vi "Add CITI Package.vi"(8 "error in (no error)":errorcluster, 10 "CITI Package":T1, 11 "CITI reference in":refnum<k24>) -> (0 "error out":errorcluster, 3 "CITI reference out":refnum<k24>)   [LabVIEW 2023, in "NI_HFNetworkAnalysis.lvlib"]
doc: "Add a CITI package in memory for the specified CITI file.\n\n<b>Note</b>\nUse <b>Save CITI File.vi</b> to write all CITI packages in memory to the referenced CITI file."
uses:
  NI_HFNetworkAnalysis.lvlib
  C:/srd-semi-rfcal-software/AuxTools/STSRFFixtureCharactUtility/Source/Code Modules/Fixture/Dependencies/HFNetworkAnalysis/Support Files/NACE.Utils.Data.dll
  Support Files/NACE.Utils.Data.dll
  Controls/CITI Package.ctl
  <vilib>/Utility/VariantDataType/VariantType.lvlib
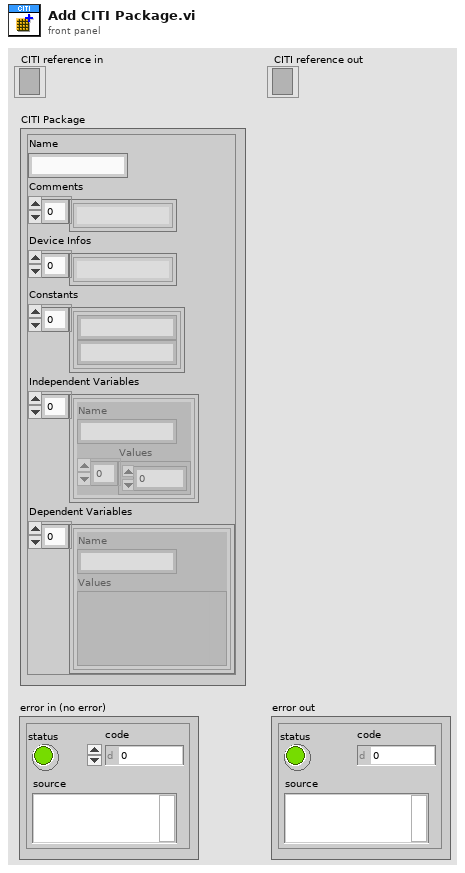
[diagram p1: front panel]
types:
  T1 = typedef "NI_HFNetworkAnalysis.lvlib/CITI Package.ctl" = cluster{"Name":string, "Comments":string[], "Device Infos":string[], "Constants":cluster{"Name":string, "Value":string}[], "Independent Variables":cluster{"Name":string, "Values":dbl[]}[], "Dependent Variables":cluster{"Name":string, "Values":variant}[]}
  T2 = typedef "VariantType.lvlib/Type.ctl" = enum8{"Invalid Type", "Void", "I8", "I16", "I32", "I64", "U8", "U16", "U32", "U64", "Single Float", "Double Float", "Extended Float", "Single Complex", "Double Complex", "Extended Complex", "Enum U8", "Enum U16", "Enum U32", "Enum U64", "Single Float With Unit", "Double Float With Unit", "Extended Float With Unit", "Single Complex with Unit", "Double Complex with Unit", "Extended Complex with Unit", "Boolean", "String", "Path", "Picture", "Tag", "Array", "Cluster", "Variant", "LV Variant", "Waveform", "Timestamp", "Digital Waveform", "Digital Data", "ExpressData", "Refnum", "External Data", "VI", "Poly VI", "LabVIEW Class Instance", "Fixed Point"}
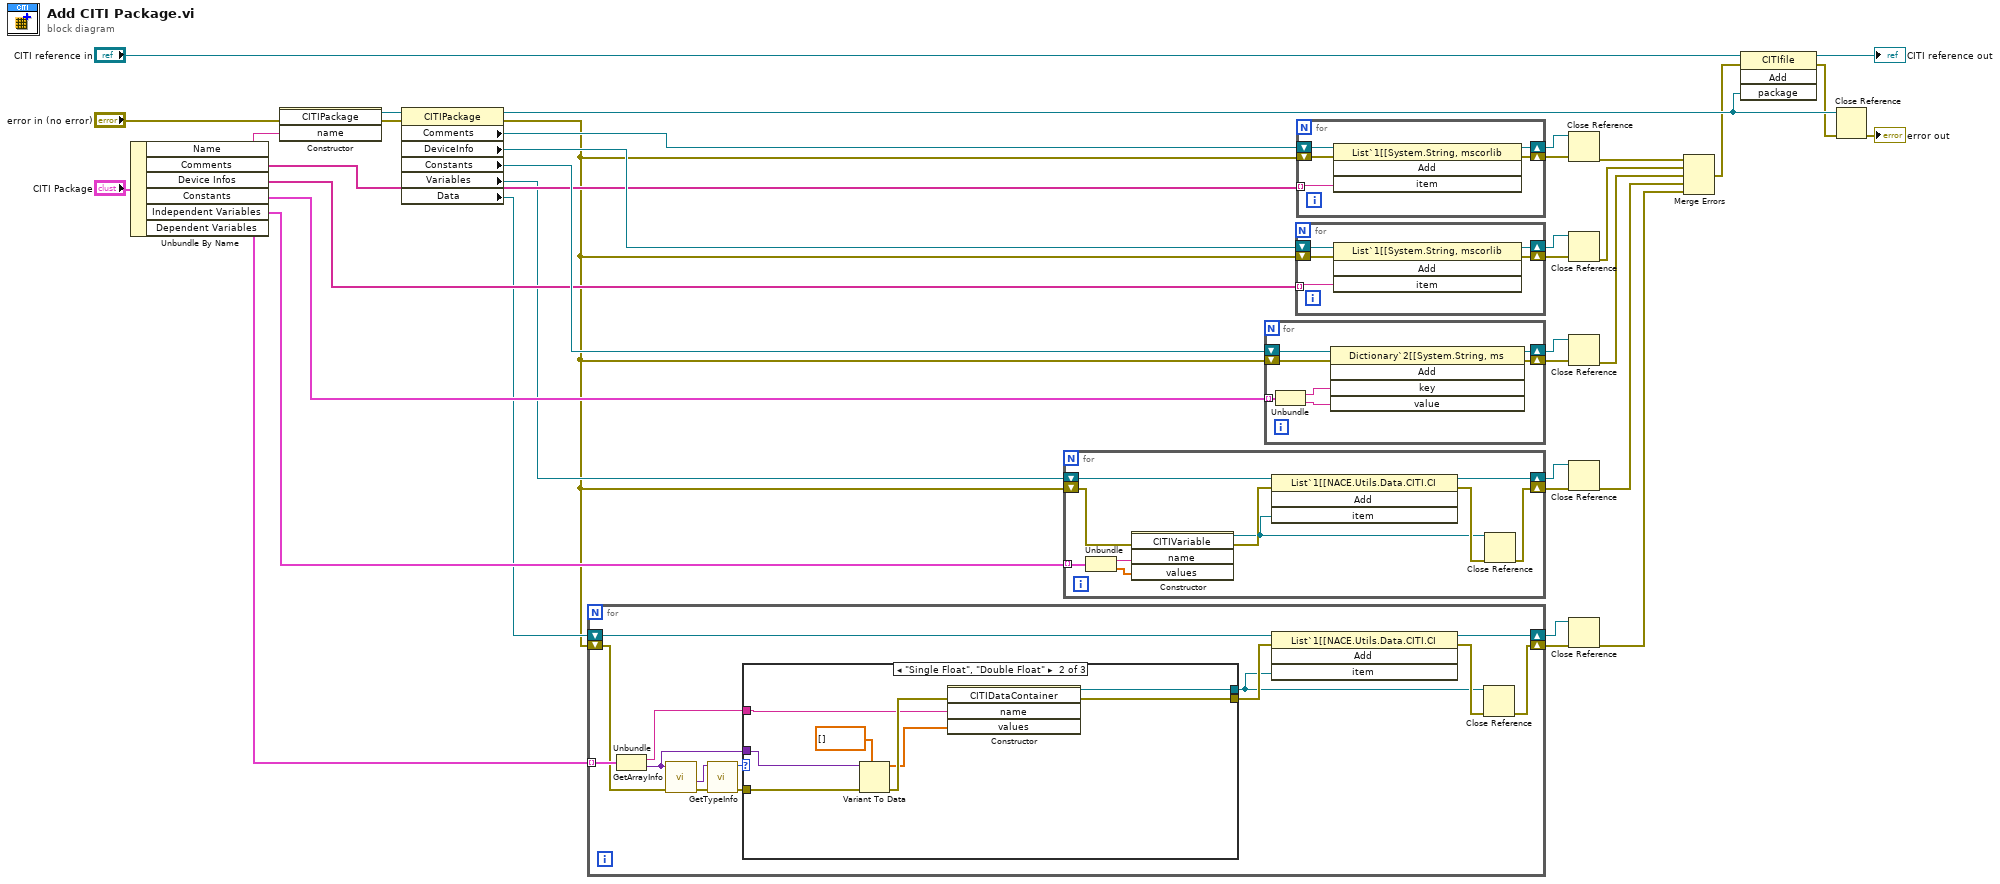
[diagram p0: block diagram]
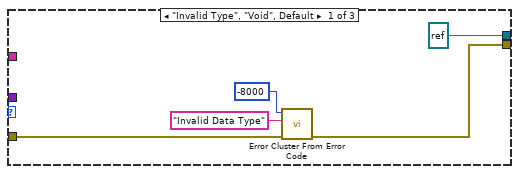
[diagram p2: hidden frame]
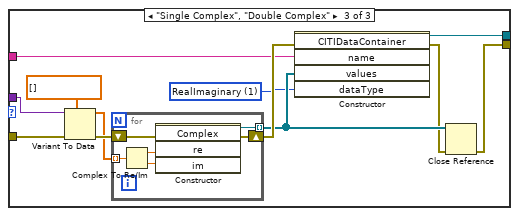
[diagram p3: hidden frame]
diagram:
  n1 = Unbundle By Name("CITI Package") -> ("Name"=w19:string, "Comments"=w18:string[], "Device Infos"=w17:string[], "Constants"=w16:cluster{"Name":string, "Value":string}[], "Independent Variables"=w15:cluster{"Name":string, "Values":dbl[]}[], "Dependent Variables"=w11:cluster{"Name":string, "Values":variant}[])
  n2 = constructor class="CITIPackage"(error in="error in (no error)", "name"=w19) -> (reference out=w35:refnum<k24>, error out=w34:errorcluster)  [unwired: 2 in, 2 out]
  n3 = property class="CITIPackage"(reference=w35, error in=w34) -> (reference out=w30:refnum<k24>, error out=w9:errorcluster, "Comments"=w33:refnum<k24>, "DeviceInfo"=w24:refnum<k24>, "Constants"=w21:refnum<k24>, "Variables"=w14:refnum<k24>, "Data"=w10:refnum<k24>)
  n4 = for {
    tunnel: w11 -> [w47] mode=indexing
    shift-right: [w48] -> w8
    shift-left: w9 -> [w39]
    shift-right: [w50] -> w7
    shift-left: w10 -> [w51]
    n5 = Unbundle(w47) -> ("Name"=w42:string, "Values"=w38:variant)
    n6 = call <vilib>:"GetArrayInfo.vi"("error in (no error)"=w39, "Variant"=w38) -> ("error out"=w44:errorcluster, "ArrayElement"=w43:variant)  [unwired: 6 in, 2 out]
    n7 = call <vilib>:"GetTypeInfo.vi"("error in (no error)"=w44, "Variant"=w43) -> ("error out"=w46:errorcluster, "Type Enum"=w45:T2)  [unwired: 5 in, 3 out]
    n8 = case shown="\"Single Float\", \"Double Float\"" w45 {
      tunnel: w46 -> [w56 w64 w75]
      tunnel: [refnum<k24> refnum ("new reference") w59 w71] -> w40
      tunnel: [w55 w60 w68] -> w41
      tunnel: w42 -> [_ w58 w67]
      tunnel: w38 -> [_ w57 w65]
      frame "Invalid Type", "Void", Default {
        n9 = call <vilib>:"Error Cluster From Error Code.vi"("error in (no error)"=w56, "error message (\"\")"="Invalid Data Type" ("error message (\"\")"), "error code (0)"=-8000) -> ("error out"=w55:errorcluster)  [unwired: 6 in]
      }
      frame "Single Float", "Double Float" {
        n10 = Variant To Data(error in=w64, type=dbl[] [], Variant=w57) -> (data=w61:dbl[], error out=w62:errorcluster)
        n11 = constructor class="CITIDataContainer"(error in=w62, "name"=w58, "values"=w61) -> (reference out=w59:refnum<k24>, error out=w60:errorcluster)  [unwired: 2 in, 3 out]
      }
      frame "Single Complex", "Double Complex" {
        w66 = 1 items=["Magnitude", "RealImaginary", "MagnitudeAngle"] ("dataType")
        n12 = Variant To Data(error in=w75, type=cdb[] [], Variant=w65) -> (data=w74:cdb[], error out=w76:errorcluster)
        n13 = for {
          tunnel: w74 -> [w79] mode=indexing
          tunnel: [w78] -> w70 mode=indexing
          shift-right: [w77] -> w72
          shift-left: w76 -> [w82]
          n14 = Complex To Re/Im(x + iy=w79) -> (x=w81:dbl, y=w80:dbl)
          n15 = constructor class="Complex"(error in=w82, "re"=w81, "im"=w80) -> (reference out=w78:refnum<k24>, error out=w77:errorcluster)  [unwired: 2 in, 3 out]
        }
        n16 = constructor class="CITIDataContainer"(error in=w72, "name"=w67, "values"=w70, "dataType"=w66) -> (reference out=w71:refnum<k24>, error out=w69:errorcluster)  [unwired: 2 in, 4 out]
        n17 = Close Reference(reference=w70, error in (no error)=w69) -> (error out=w68:errorcluster)
      }
    }
    n18 = invoke class="List`1[[NACE.Utils.Data.CITI.CI" method="Add"(reference=w51, error in=w41, "item"=w40) -> (reference out=w50:refnum<k24>, error out=w49:errorcluster)  [unwired: 1 in, 2 out]
    n19 = Close Reference(reference=w40, error in (no error)=w49) -> (error out=w48:errorcluster)
  }
  n20 = for {
    tunnel: w15 -> [w92] mode=indexing
    shift-right: [w85] -> w12
    shift-left: w14 -> [w89]
    shift-right: [w84] -> w13
    shift-left: w9 -> [w83]
    n21 = Unbundle(w92) -> ("Name"=w91:string, "Values"=w90:dbl[])
    n22 = constructor class="CITIVariable"(error in=w83, "name"=w91, "values"=w90) -> (reference out=w86:refnum<k24>, error out=w88:errorcluster)  [unwired: 2 in, 3 out]
    n23 = invoke class="List`1[[NACE.Utils.Data.CITI.CI" method="Add"(reference=w89, error in=w88, "item"=w86) -> (reference out=w85:refnum<k24>, error out=w87:errorcluster)  [unwired: 1 in, 2 out]
    n24 = Close Reference(reference=w86, error in (no error)=w87) -> (error out=w84:errorcluster)
  }
  n25 = for {
    shift-right: [w97] -> w23
    shift-left: w9 -> [w98]
    shift-right: [w96] -> w22
    shift-left: w21 -> [w99]
    tunnel: w16 -> [w93] mode=indexing
    n26 = Unbundle(w93) -> ("Name"=w95:string, "Value"=w94:string)
    n27 = invoke class="Dictionary`2[[System.String, ms" method="Add"(reference=w99, error in=w98, "key"=w95, "value"=w94) -> (reference out=w96:refnum<k24>, error out=w97:errorcluster)  [unwired: 1 in, 3 out]
  }
  n28 = for {
    tunnel: w17 -> [w103] mode=indexing
    shift-right: [w101] -> w26
    shift-left: w9 -> [w102]
    shift-right: [w100] -> w25
    shift-left: w24 -> [w104]
    n29 = invoke class="List`1[[System.String, mscorlib" method="Add"(reference=w104, error in=w102, "item"=w103) -> (reference out=w100:refnum<k24>, error out=w101:errorcluster)  [unwired: 1 in, 2 out]
  }
  n30 = for {
    tunnel: w18 -> [w108] mode=indexing
    shift-right: [w106] -> w28
    shift-left: w9 -> [w107]
    shift-right: [w105] -> w27
    shift-left: w33 -> [w109]
    n31 = invoke class="List`1[[System.String, mscorlib" method="Add"(reference=w109, error in=w107, "item"=w108) -> (reference out=w105:refnum<k24>, error out=w106:errorcluster)  [unwired: 1 in, 2 out]
  }
  n32 = Close Reference(reference=w27, error in (no error)=w28) -> (error out=w6:errorcluster)
  n33 = Close Reference(reference=w25, error in (no error)=w26) -> (error out=w5:errorcluster)
  n34 = Close Reference(reference=w22, error in (no error)=w23) -> (error out=w4:errorcluster)
  n35 = Close Reference(reference=w12, error in (no error)=w13) -> (error out=w3:errorcluster)
  n36 = Close Reference(reference=w7, error in (no error)=w8) -> (error out=w2:errorcluster)
  n37 = Merge Errors(w6, w5, w4, w3, w2) -> (w1:errorcluster)
  n38 = invoke class="CITIfile" method="Add"(reference="CITI reference in", error in=w1, "package"=w30) -> (reference out=→"CITI reference out":refnum<k24>, error out=w29:errorcluster)  [unwired: 1 in, 2 out]
  n39 = Close Reference(reference=w30, error in (no error)=w29) -> (error out=→"error out":errorcluster)
